vi "Build Full Directory Path.vi"(2 "Parent Directory":string, 3 "Sub Directory":string) -> (0 "Full Directory Path":string)   [LabVIEW 2020, in "AoC 2022.lvlib"]
uses:
  AoC 2022.lvlib
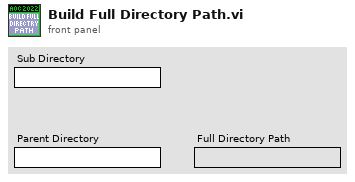
[diagram p1: front panel]
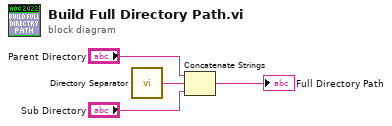
[diagram p0: block diagram]
diagram:
  n1 = call "Directory Separator.vi"() -> ("Directory Separator"=w2:string)
  n2 = Concatenate Strings("Parent Directory", w2, "Sub Directory") -> (→"Full Directory Path":string)
